vi "write csi (host with fpga).vi"(5 "channel num":u32=1, 6 "trigger to write csi":bool, 7 "csi per packet":u32=242, 9 "number of packets to detect":u32, 10 "file ref":refnum<file>, 11 "fpga cluster":T1 {"Daughterboard Clock Rate" format="%#.3pHz"; "FPGA Data Clock Rate" format="%#.3pHz"; "Data Clock Rate" format="%#.3pHz"; "Characterization Data"."Frequencies [Hz]" format="%#_6p"; "EEPROM Characterization Header"."Pointer to Device Data Header" format="%x"; "EEPROM Characterization Header"."Checksum" format="%x"; "Device Data Header"."Pointer to Characterization Data" format="%x"; "Device Data Header"."Checksum" format="%x"; "EEPROM Header"."Pointer to User Header" format="%x"; "EEPROM Header"."Pointer to Factory Header" format="%x"; "EEPROM Header"."Product Code" format="%x"; "EEPROM Header"."Checksum" format="%x"}) -> (1 "csi num":u32, 2 "csi is written":bool, 3 "csi":string)   [LabVIEW 2020]
uses:
  <instrlib>/niUsrpRio/Config/v1/Host/Public/niUsrpRio Session.ctl
  <instrlib>/_niInstr/Register Bus/v0/Host/Public/Register Bus Session.ctl
  <instrlib>/_niInstr/Register Bus/v0/Host/Private/Session Data.ctl
  <instrlib>/niUsrpRio/Config/v1/Host/Private/DB Queue Reference.ctl
  <instrlib>/niUsrpRio/Config/v1/Host/Private/Daughterboard Data.ctl
  <instrlib>/niUsrpRio/Config/v1/Host/Private/ATR state data.ctl
  <instrlib>/niUsrpRio/Config/v1/Host/Private/Antenna Configuration.ctl
  <instrlib>/niUsrpRio/Config/v1/Host/Private/CPLD Power Mode.ctl
  <instrlib>/niUsrpRio/Config/v1/Host/Public/EEPROM Header.ctl
  <instrlib>/niUsrpRio/Config/v1/Host/Public/EEPROM Device Data Header.ctl
  <instrlib>/niUsrpRio/Config/v1/Host/Public/EEPROM Characterization Header.ctl
  <instrlib>/niUsrpRio/Config/v1/Host/Public/Characterization Data.ctl
  <instrlib>/niUsrpRio/Config/v1/Host/Public/IQ Imbalance.ctl
  Host/SubVIs/Streaming Xvcr FPGA Ref.ctl
  <vilib>/rvi/interface/common/niFpgaWaitOnOcc.vi
  <vilib>/Utility/error.llb/Error Cluster From Error Code.vi
  <vilib>/rvi/errors/niLvFpgaAdjustHostInterfaceError.vi
  <vilib>/rvi/interface/nirviMethod/nirviMethod.xnode
  <vilib>/FPGAPlugInAG/Dynamic/niLvFpga_ReadFifo_Dynamic.vi
  <vilib>/rvi/errors/niLvFpgaMergeErrorWithErrorCode.vi
  <vilib>/FPGAPlugInAG/Dynamic/niLvFpga_ConfigureFifo_Dynamic.vi
  <instrlib>/niUsrpRio/Config/v1/Host/niUsrpRio Config v1 Host.lvlib
  <instrlib>/_niInstr/Register Bus/v0/Host/niInstr Register Bus v0 Host.lvlib
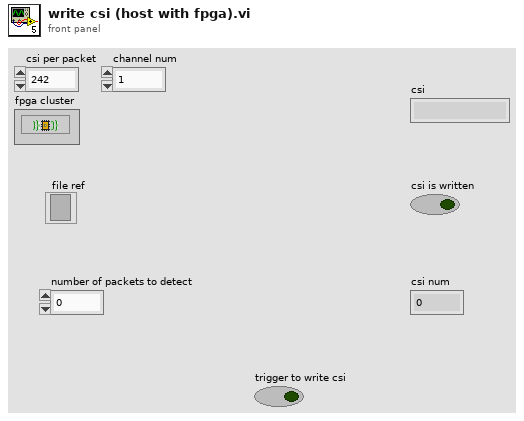
[diagram p1: front panel]
types:
  T1 = typedef "niUsrpRio Config v1 Host.lvlib/niUsrpRio Session.ctl" = cluster{"FPGA Interface":refnum<k20>, "RIO Interface Number":u32, "Data Clock Rate":u32, "FPGA Data Clock Rate":u32, "Global Settings Register Bus":T2, "Radio 0 Settings Register Bus":T2, "Radio 1 Settings Register Bus":T2, "Radio Settings Bus Semaphore":T3, "DB Queues":T4[], "Characterization Data Valid?":bool, "EEPROM Header":T5, "Device Data Header":T6, "EEPROM Characterization Header":T7, "Characterization Data":T8[], "FPGA Current Version":u32, "FPGA Oldest Compatible Version":u32, "Fixed Logic Current Version":u32, "Fixed Logic Oldest Compatible Version":u32, "FPGA Radio Settings Bus Current Version":u32, "FPGA Radio Settings Bus Oldest Compatible Version":u32, "FPGA Board Config Current Version":u32, "FPGA Board Config Oldest Compatible Version":u32, "Daughterboard Clock Rate":u32, "daughterboard configuration session handles":u64[]}
  T2 = typedef "niInstr Register Bus v0 Host.lvlib/Register Bus Session.ctl" = refnum<queue>
  T3 = typedef "Semaphore RefNum" = refnum<k1>
  T4 = typedef "niUsrpRio Config v1 Host.lvlib/DB Queue Reference.ctl" = refnum<queue>
  T5 = typedef "niUsrpRio Config v1 Host.lvlib/EEPROM Header.ctl" = cluster{"Checksum":u32, "Product Code":u16, "Hardware Current Version":u16, "Hardware Oldest Compatible Version":u16, "EEPROM Map Current Version":u16, "EEPROM Map Oldest Compatible Version":u16, "User Password":string, "Pointer to Factory Header":u32, "Pointer to User Header":u32, "Recommended Interval":u16, "Number of Reserved Bytes":i32, "Number of Daughterboards":u8, "Daughterboard IDs":u16[], "Daughterboard Serial Numbers":string[]}
  T6 = typedef "niUsrpRio Config v1 Host.lvlib/EEPROM Device Data Header.ctl" = cluster{"Checksum":u32, "Number of Channels":u8, "Number of Gain Settings":u16[], "Pointer to Characterization Data":u32[], "Number of Reserved Bytes":i32, "Number of Frequencies":u16[]}
  T7 = typedef "niUsrpRio Config v1 Host.lvlib/EEPROM Characterization Header.ctl" = cluster{"Checksum":u32, "Date":timestamp, "Temperature":sgl, "Misc. Info":string, "Pointer to Device Data Header":u32, "Number of Reserved Bytes":i32}
  T8 = typedef "niUsrpRio Config v1 Host.lvlib/Characterization Data.ctl" = cluster{"Gains[dB]":dbl[], "Frequencies [Hz]":dbl[], "IQ Imbalance Table":T9[], "Measured Gains[dB]":dbl[][]}
  T9 = typedef "niUsrpRio Config v1 Host.lvlib/IQ Imbalance.ctl" = cluster{"Gain Imbalance [linear]":dbl, "Phase Imbalance [radians]":dbl, "Offset":cdb}
  T10 = typedef "Streaming Xvcr FPGA Ref.ctl" = refnum<k20>
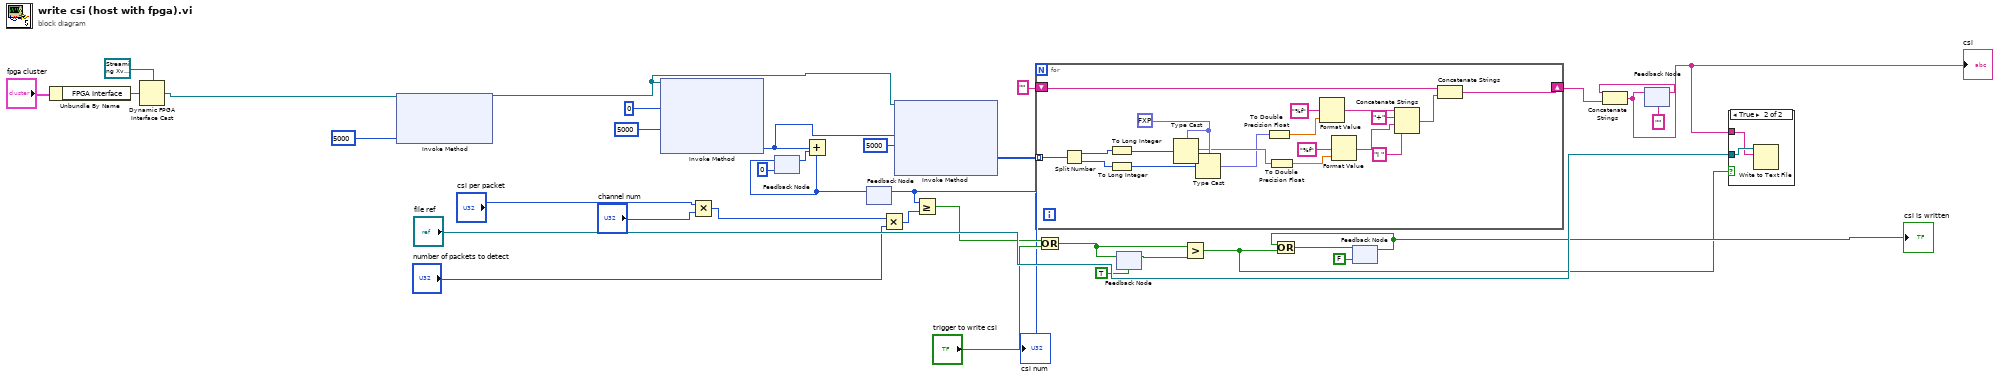
[diagram p0: block diagram]
diagram:
  n1 = Unbundle By Name("fpga cluster") -> ("FPGA Interface"=w4:refnum<k20>)
  n2 = Dynamic FPGA Interface Cast(Session In=T10 refnum ("Type"), Type=w4) -> (Session Out=w1:T10)
  n3 = xnode "Invoke Method"("FPGA VI Reference In"=w1, "Requested Depth"=u32 5000) -> ("FPGA VI Reference Out"=w5:T10)  [unwired: 1 in, 2 out]
  n4 = xnode "Invoke Method"("FPGA VI Reference In"=w5, "Number of Elements"=u32 0, "Timeout (ms)"=5000) -> ("Elements Remaining"=w19:u32)  [unwired: 1 in, 3 out]
  n5 = Multiply(x="csi per packet", y="channel num") -> (x*y=w8:u32)
  n6 = feedback #1(u32 0) -> (w20:u32)
  n7 = Add(x=w19, y=w20) -> (x+y=w22:u32)
  n8 = feedback-in #1(w22) -> ()
  n9 = feedback #2() -> (w23:u32)  [unwired: 1 in]
  "csi num" <- w23
  n10 = feedback-in #2(w22) -> ()
  n11 = Multiply(x=w8, y="number of packets to detect") -> (x*y=w24:u32)
  n12 = xnode "Invoke Method"("FPGA VI Reference In"=w5, "Number of Elements"=w19, "Timeout (ms)"=5000) -> ("Data"=w16:u64[])  [unwired: 1 in, 3 out]
  n13 = Greater Or Equal?(x=w23, y=w24) -> (x >= y?=w32:bool)
  n14 = for {
    tunnel: w16 -> [w41] mode=indexing
    shift-right: [w36] -> w17
    shift-left: "" -> [w38]
    w51 = fxp<+/-,32,11> 0.0 ("Number of Elements")
    n15 = Split Number(x=w41) -> (hi(x)=w54:u32, lo(x)=w53:u32)
    n16 = To Long Integer(number=w54) -> (32bit integer=w52:i32)
    n17 = To Long Integer(number=w53) -> (32bit integer=w40:i32)
    n18 = Type Cast(type=w51, x=w52) -> (*(type *) &x=w49:fxp<+/-,32,11>)
    n19 = Type Cast(type=w51, x=w40) -> (*(type *) &x=w39:fxp<+/-,32,11>)
    n20 = To Double Precision Float(number=w39) -> (double precision float=w48:dbl)
    n21 = To Double Precision Float(number=w49) -> (double precision float=w46:dbl)
    n22 = Format Value(format string="%f", value (0)=w48) -> (output string=w45:string)  [unwired: 1 in]
    n23 = Format Value(format string="%f", value (0)=w46) -> (output string=w43:string)  [unwired: 1 in]
    n24 = Concatenate Strings(w45, "+" ("string"), w43, "i " ("string")) -> (w37:string)
    n25 = Concatenate Strings(w38, w37) -> (w36:string)
  }
  n26 = Or(x=w32, y="trigger to write csi") -> (x .or. y?=w29:bool)
  n27 = feedback #3(TRUE ("trigger to write csi and samples")) -> (w27:bool)
  n28 = feedback-in #3(w29) -> ()
  n29 = Greater?(x=w29, y=w27) -> (0:w33:bool)
  n30 = feedback #4(FALSE) -> (w34:bool)
  "csi is written" <- w34
  n31 = Or(x=w34, y=w33) -> (x .or. y?=w31:bool)
  n32 = feedback-in #4(w31) -> ()
  n33 = feedback #5("" ("output string")) -> (w14:string)
  n34 = Concatenate Strings(w14, w17) -> (w15:string)
  "csi" <- w15
  n35 = feedback-in #5(w15) -> ()
  n36 = case shown="True" w33 {
    tunnel: "file ref" -> [_ w56]
    tunnel: w15 -> [_ w55]
    frame False {
    }
    frame True {
      n37 = Write to Text File(file (use dialog)=w56, text=w55) -> ()  [unwired: 2 in, 3 out]
    }
  }
